vi "FitParabola2 (SubVI).vi"(0 "x values":dbl[](array[numeric]), 1 "y values":dbl[](array[numeric]), 2 "delta y values":dbl[](array[numeric]), 3 "confidence level":dbl=0.95, 5 "error in":errorcluster, 6 "Use all points":bool, 7 "Estimated minimum":dbl, 8 "Poly fit algorithm":T2 items=["SVD", "Givens", "Givens2", "Householder", "LU Decomposition", "Cholesky", "SVD for Rank Deficient H"], 9 "Estimated width":dbl, 10 "Polynomial Coefficient Constraint":cluster{"order":i32, "coefficient":dbl}[](array[cluster]), 11 "Nsigma Low":dbl=4.0 format="%#_13g", 12 "Minimization inputs":T1={"Minimizing alg"=0, "Search start"=0.0, "Search end"=1.0, "Search accuracy"=1e-08, "Step type"=0} {"Step type" items=["fixed function", "modified function"]; "Search accuracy" format="%.2e"; "Search end" format="%.2f"; "Search start" format="%.2f"; "Minimizing alg" items=["Golden Section Search", "Brent with Derivatives"]}, 13 "Nsigma High":dbl=4.0 format="%#_13g") -> (14 "Plot with quadratic fit":T3(graph), 15 "Minima":dbl[](array[numeric]) format="%.2f", 16 "Uncertainty on minimum":dbl, 19 "error out":errorcluster)   [LabVIEW 2016]
uses:
  <vilib>/Analysis/6fits.llb/General Linear Fit Algorithm.ctl
  <vilib>/Analysis/6fits.llb/Confidence Interval (Polynomial).vi
  <vilib>/Analysis/NI_AALPro.lvlib
  <vilib>/gmath/NI_Gmath.lvlib
panel:
  out "Delta Polynomial Coefficients":dbl[](array[numeric])
  out "Fitted quadratic":string
  out "f(Minima)":dbl[](array[numeric]) format="%.2f"
  out "Selected delta y values":dbl[](array[numeric])
  out "Best Quadratic Fit":dbl[](array[numeric])
  out "Poly fit residue":dbl
  out "Selected y values":dbl[](array[numeric])
  out "Selected x values":dbl[](array[numeric])
  out "Polynomial Coefficients":dbl[](array[numeric])
  # "RESULTS"
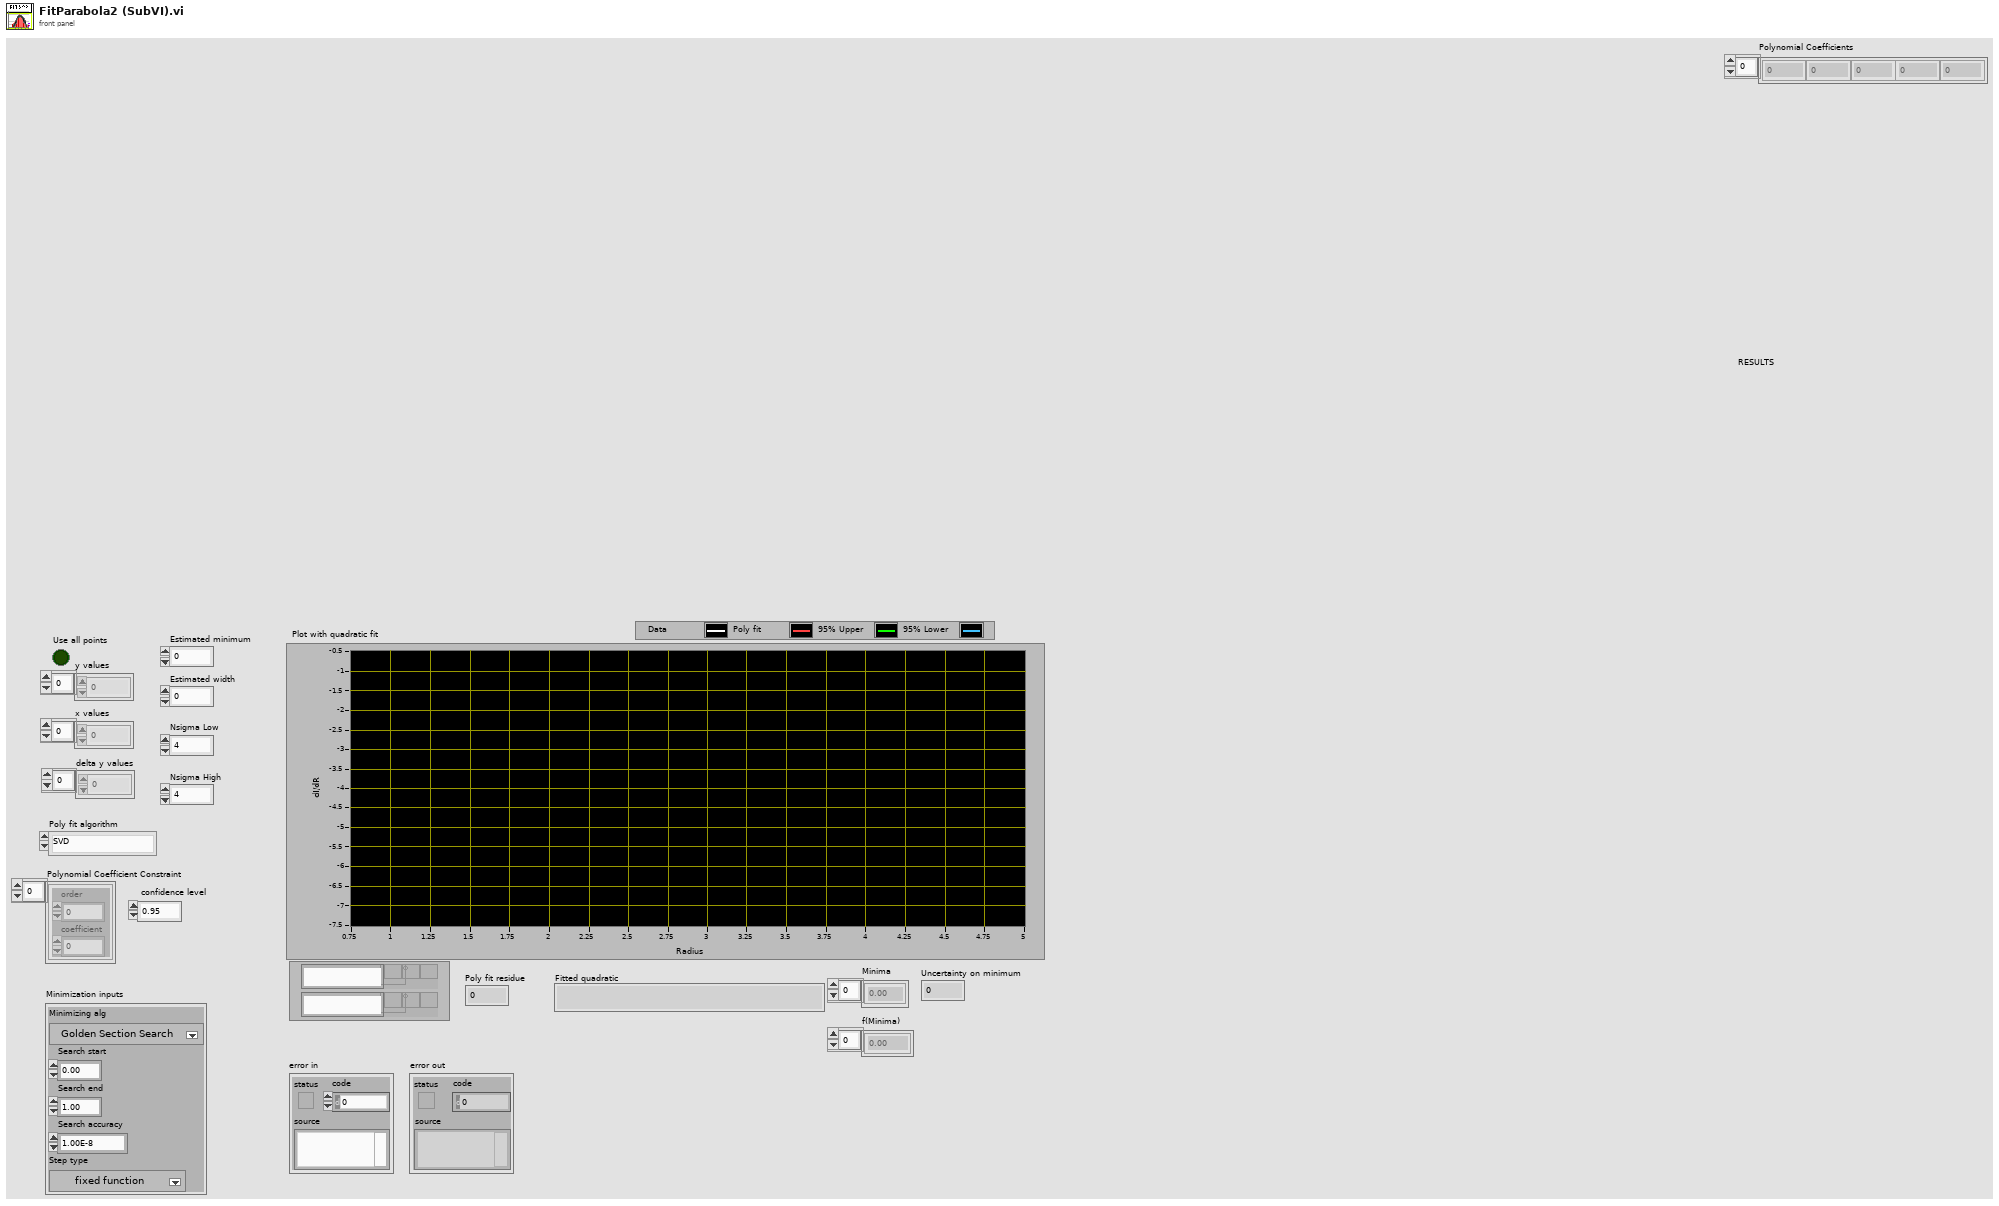
[diagram p1: front panel]
types:
  T1 = cluster{"Minimizing alg":u16, "Search start":dbl, "Search end":dbl, "Search accuracy":dbl, "Step type":u16}
  T2 = typedef "NI_AALPro.lvlib/General Linear Fit Algorithm.ctl" = u16
  T3 = cluster{"Radius bins":dbl[], "Best Gaussian Fit":dbl[]}[]
  T4 = cluster{"Selected x values":dbl[], "Selected y values":dbl[]}
  T5 = cluster{"Selected x values":dbl[], "Best Quadratic Fit":dbl[]}
  T6 = cluster{"Selected x values":dbl[], "Upper Bound":dbl[]}
  T7 = cluster{"Selected x values":dbl[], "Lower Bound":dbl[]}
  T8 = cluster{"Selected x values":dbl[], "Lower Bound":dbl[]}[]
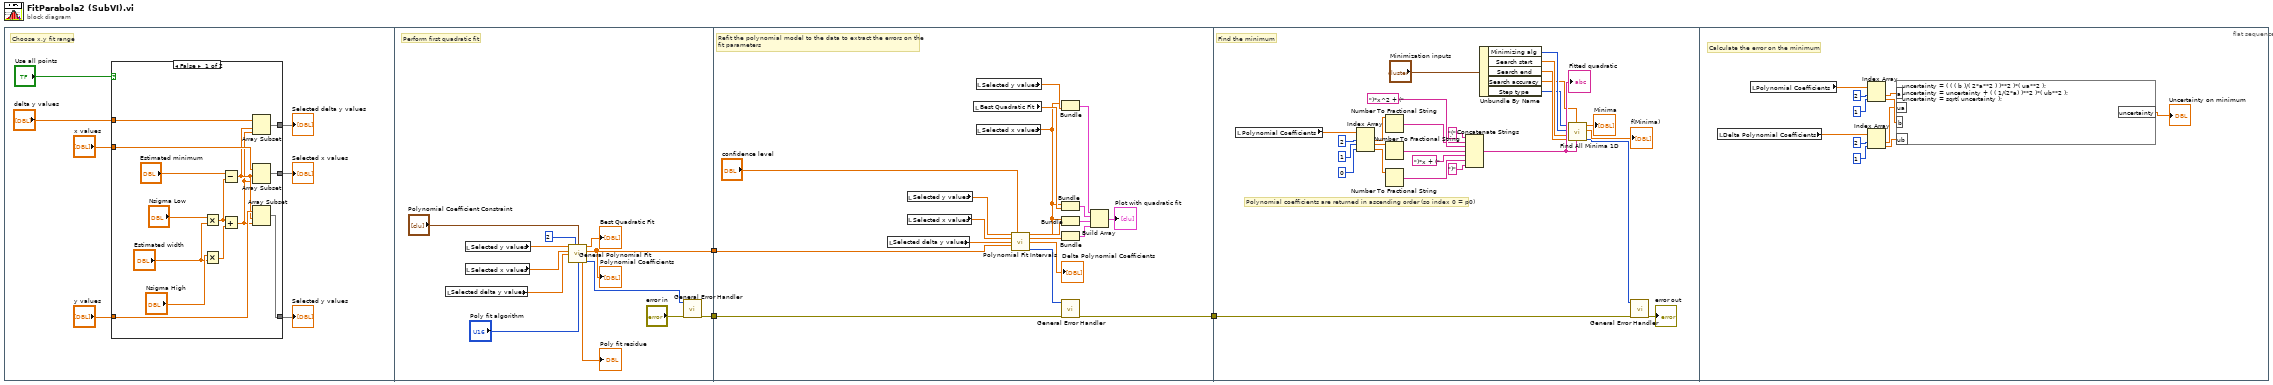
[diagram p0: block diagram]
diagram:
  n1 = flat-sequence {
    tunnel: [w34] -> w3
    tunnel: [w28] -> w2
    tunnel: w3 -> [w44]
    tunnel: w2 -> [w42]
    tunnel: [w41] -> w1
    tunnel: w1 -> [w65]
    frame #0 {
      # "Choose x,y fit range"
      n2 = case shown="False" "Use all points" {
        tunnel: "y values" -> [w22 w26]
        tunnel: [w21 w26] -> w6
        tunnel: "x values" -> [w20 w27]
        tunnel: [w19 w27] -> w7
        tunnel: "delta y values" -> [w14 w25]
        tunnel: [w11 w25] -> w4
        frame False {
          n3 = Multiply(x="Nsigma Low", y="Estimated width") -> (x*y=w16:dbl)
          n4 = Multiply(x="Nsigma High", y="Estimated width") -> (x*y=w15:dbl)
          n5 = Subtract(x="Estimated minimum", y=w16) -> (x-y=w13:dbl)
          n6 = Add(x=w16, y=w15) -> (x+y=w12:dbl)
          n7 = Array Subset(array=w14, index=w13, length=w12) -> (w11:dbl[])
          n8 = Array Subset(array=w20, index=w13, length=w12) -> (w19:dbl[])
          n9 = Array Subset(array=w22, index=w13, length=w12) -> (w21:dbl[])
        }
        frame True {
        }
      }
      "Selected y values" <- w6
      "Selected x values" <- w7
      "Selected delta y values" <- w4
    }
    frame #1 {
      # "Perform first quadratic fit"
      n10 = local read "Selected delta y values"() -> (w29:dbl[])
      n11 = local read "Selected y values"() -> (w39:dbl[])
      n12 = local read "Selected x values"() -> (w38:dbl[])
      n13 = call <vilib>:"General Polynomial Fit.vi"("Y"=w39, "polynomial order"=2, "Coefficient Constraint"="Polynomial Coefficient Constraint", "X"=w38, "Weight"=w29, "algorithm"="Poly fit algorithm") -> ("Best Polynomial Fit"=→"Best Quadratic Fit":dbl[], "Polynomial Coefficients"=w28:dbl[], "residue"=→"Poly fit residue":dbl, "error"=w35:i32)  [unwired: 6 in]
      "Polynomial Coefficients" <- w28
      n14 = call <vilib>:"General Error Handler.vi"("[error code] (0)"=w35, "error in (no error)"="error in") -> ("error out"=w34:errorcluster)  [unwired: 9 in, 4 out]
    }
    frame #2 {
      # "Refit the polynomial model to the data to extract the errors on the\nfit parameters"
      n15 = local read "Selected delta y values"() -> (w43:dbl[])
      n16 = local read "Selected y values"() -> (w58:dbl[])
      n17 = local read "Selected x values"() -> (w57:dbl[])
      n18 = local read "Best Quadratic Fit"() -> (w54:dbl[])
      n19 = local read "Selected y values"() -> (w55:dbl[])
      n20 = local read "Selected x values"() -> (w50:dbl[])
      n21 = call-poly <vilib>:"Polynomial Fit Intervals.vi"("Y"=w58, "confidence level"="confidence level", "X"=w57, "Weight"=w43, "Polynomial Coefficients"=w42) -> ("Upper Bound"=w52:dbl[], "Lower Bound"=w51:dbl[], "Delta Polynomial Coefficients"=→"Delta Polynomial Coefficients":dbl[], "error"=w45:i32)  [unwired: 7 in]
      n22 = Bundle("Selected x values"=w50, "Selected y values"=w55) -> (w53:T4)  [unwired: 1 in]
      n23 = Bundle("Selected x values"=w50, "Best Quadratic Fit"=w54) -> (w49:T5)  [unwired: 1 in]
      n24 = Bundle("Selected x values"=w50, "Upper Bound"=w52) -> (w48:T6)  [unwired: 1 in]
      n25 = Bundle("Selected x values"=w50, "Lower Bound"=w51) -> (w47:T7)  [unwired: 1 in]
      n26 = call <vilib>:"General Error Handler.vi"("[error code] (0)"=w45, "error in (no error)"=w44) -> ("error out"=w41:errorcluster)  [unwired: 9 in, 4 out]
      n27 = Build Array(w53, w49, w48, w47) -> (→"Plot with quadratic fit":T8)
    }
    frame #3 {
      # "Polynomial coefficients are returned in ascending order (so index 0 = p0)"
      # "Find the minimum"
      n28 = local read "Polynomial Coefficients"() -> (w68:dbl[])
      n29 = Index Array(array=w68, index #1=2 ("index"), index #2=1 ("index"), index #3=0 ("index")) -> (element #1=w69:dbl, element #2=w70:dbl, element #3=w71:dbl)
      n30 = Number To Fractional String(number=w69) -> (F-format string=w77:string)  [unwired: 3 in]
      n31 = Number To Fractional String(number=w70) -> (F-format string=w76:string)  [unwired: 3 in]
      n32 = Number To Fractional String(number=w71) -> (F-format string=w75:string)  [unwired: 3 in]
      n33 = Concatenate Strings("(" ("string"), w77, ")*x^2 + (" ("string"), w76, ")*x + (" ("string"), w75, ")" ("string")) -> (w82:string)
      "Fitted quadratic" <- w82
      n34 = Unbundle By Name("Minimization inputs") -> ("Minimizing alg"=w64:u16, "Search start"=w63:dbl, "Search end"=w62:dbl, "Search accuracy"=w61:dbl, "Step type"=w60:u16)
      n35 = call <vilib>:"Find All Minima 1D.vi"("formula"=w82, "accuracy"=w61, "end"=w62, "start"=w63, "algorithm"=w64, "step type"=w60) -> ("error"=w67:i32, "f(Minima)"=→"f(Minima)":dbl[], "Minima"=→"Minima":dbl[])  [unwired: 1 out]
      n36 = call <vilib>:"General Error Handler.vi"("[error code] (0)"=w67, "error in (no error)"=w65) -> ("error out"=→"error out":errorcluster)  [unwired: 9 in, 4 out]
    }
    frame #4 {
      # "Calculate the error on the minimum"
      n37 = local read "Delta Polynomial Coefficients"() -> (w95:dbl[])
      n38 = local read "Polynomial Coefficients"() -> (w92:dbl[])
      n39 = Index Array(array=w92, index #1=2 ("index"), index #2=1 ("index")) -> (element #1=w89:dbl, element #2=w88:dbl)
      n40 = Index Array(array=w95, index #1=2 ("index"), index #2=1 ("index")) -> (element #1=w87:dbl, element #2=w86:dbl)
      n41 = formula code="uncertainty = ( ( ( b )/( 2*a**2 ) )**2 )*( ua**2 );\nuncertainty = uncertainty + ( ( 1/(2*a) )**2 )*( ub**2 ); \nuncertainty = sqrt( uncertainty );"("a"=w89, "b"=w88, "ua"=w87, "ub"=w86) -> ("uncertainty"=→"Uncertainty on minimum":dbl)
    }
  }
